vi "FPGA_Main.vi"() -> ()   [LabVIEW 2017]
doc: "Przekazywanie sygnału audio, o wybranej częstotliwości próbkowania, do FIFO. Vi ma za zadanie przeprowadzić pierwszą selekcję sygnałów, poprzez wprowadzenie odpowiedniego \"Thresholdu\", a następnie zebrania odpowiedniej ilości próbek, aby wysłać paczkę do RT."
uses:
  Custom Controls/#typedef_MicrophoneData.ctl
  <vilib>/LabVIEW Targets/FPGA/RIO/BlueMoonOnboardIO/nicrio_cRIO-BlueMoonOnboardAi_TerminalMod.ctl
  <vilib>/LabVIEW Targets/FPGA/RIO/BlueMoonOnboardIO/nicrio_cRIO-BlueMoonOnboardAi_VoltageRange.ctl
  <vilib>/rvi/Emulation/niFpgaGetClockAttributes.vi
  <vilib>/rvi/Emulation/niFpgaSctlEmulationGetInTimedLoop.vi
  <vilib>/rvi/Emulation/niFpgaEmulationReportErrorSimple.vi
  <vilib>/rvi/eio/common/nirviEmuTemplateMethod_errors.vi
  <vilib>/rvi/eio/common/nirviEmuTemplatePropertySet_noerrors.vi
  <vilib>/rvi/interface/RandomDataEmulation/niFpgaRandomDataHandleErrors.vi
  <vilib>/rvi/Emulation/niFpgaCriticalErrorInLSC.vi
  <vilib>/eio/EIONode/EIONode.xnode
  <vilib>/eio/EIOPropertyNode/EIOPropertyNode.xnode
  <vilib>/rvi/Analysis/measure/butterworth/XNode/niFpgaButterworthFilter.xnode
  <vilib>/rvi/DataTransferAndStorage/Container/XNode/niFpgaContainer.xnode
  <vilib>/rvi/interface/RandomDataEmulation/nirviRandomDataFpgaReadWriteTemplate.vi
  <vilib>/rvi/eio/common/nirviEmuTemplatePropertyGet_errors.vi
  <vilib>/rvi/eio/common/nirviEmuTemplatePropertyGet_noerrors.vi
  <vilib>/rvi/eio/common/nirviEmuTemplatePropertySet_errors.vi
panel:
  in  "SamplesToSend":u32
  in  "NoiseSamplesToReject":u32
  in  "Threshold":fxp<+/-,28,9>
  out "Mic_4_FIFO_Timed Out?":bool
  out "Mic_3_FIFO_Timed Out?":bool
  out "Mic_2_FIFO_Timed Out?":bool
  out "Mic_1_FIFO_Timed Out?":bool
  in  "AcqLoopDelay(uSec)":u32 caption="Count(uSec)"
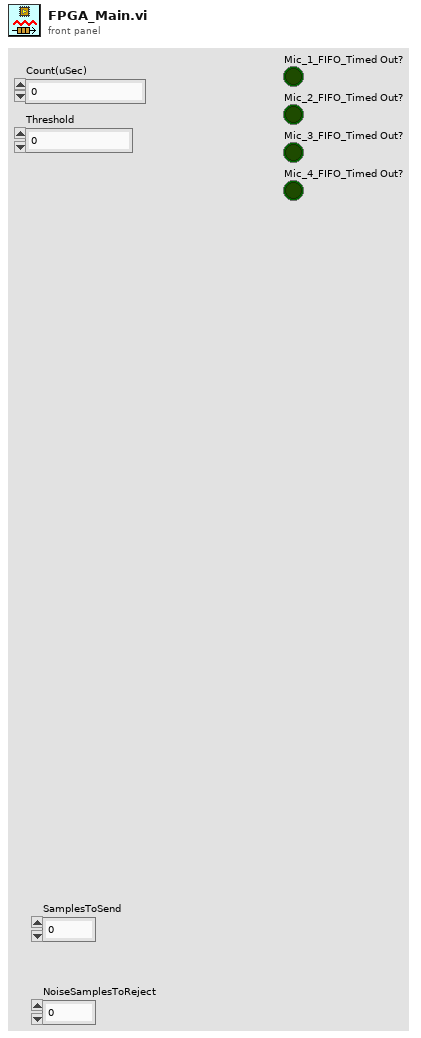
[diagram p1: front panel]
types:
  T1 = typedef "#typedef_MicrophoneData.ctl" = cluster{"output data":fxp<+/-,28,9>, "output data":fxp<+/-,28,9>, "output data":fxp<+/-,28,9>, "output data":fxp<+/-,28,9>}
  T2 = typedef "nicrio_cRIO-BlueMoonOnboardAi_VoltageRange.ctl" = u8
  T3 = typedef "nicrio_cRIO-BlueMoonOnboardAi_TerminalMod.ctl" = u8
  T4 = cluster{"output data":bool, "output data":bool, "output data":bool, "output data":bool}
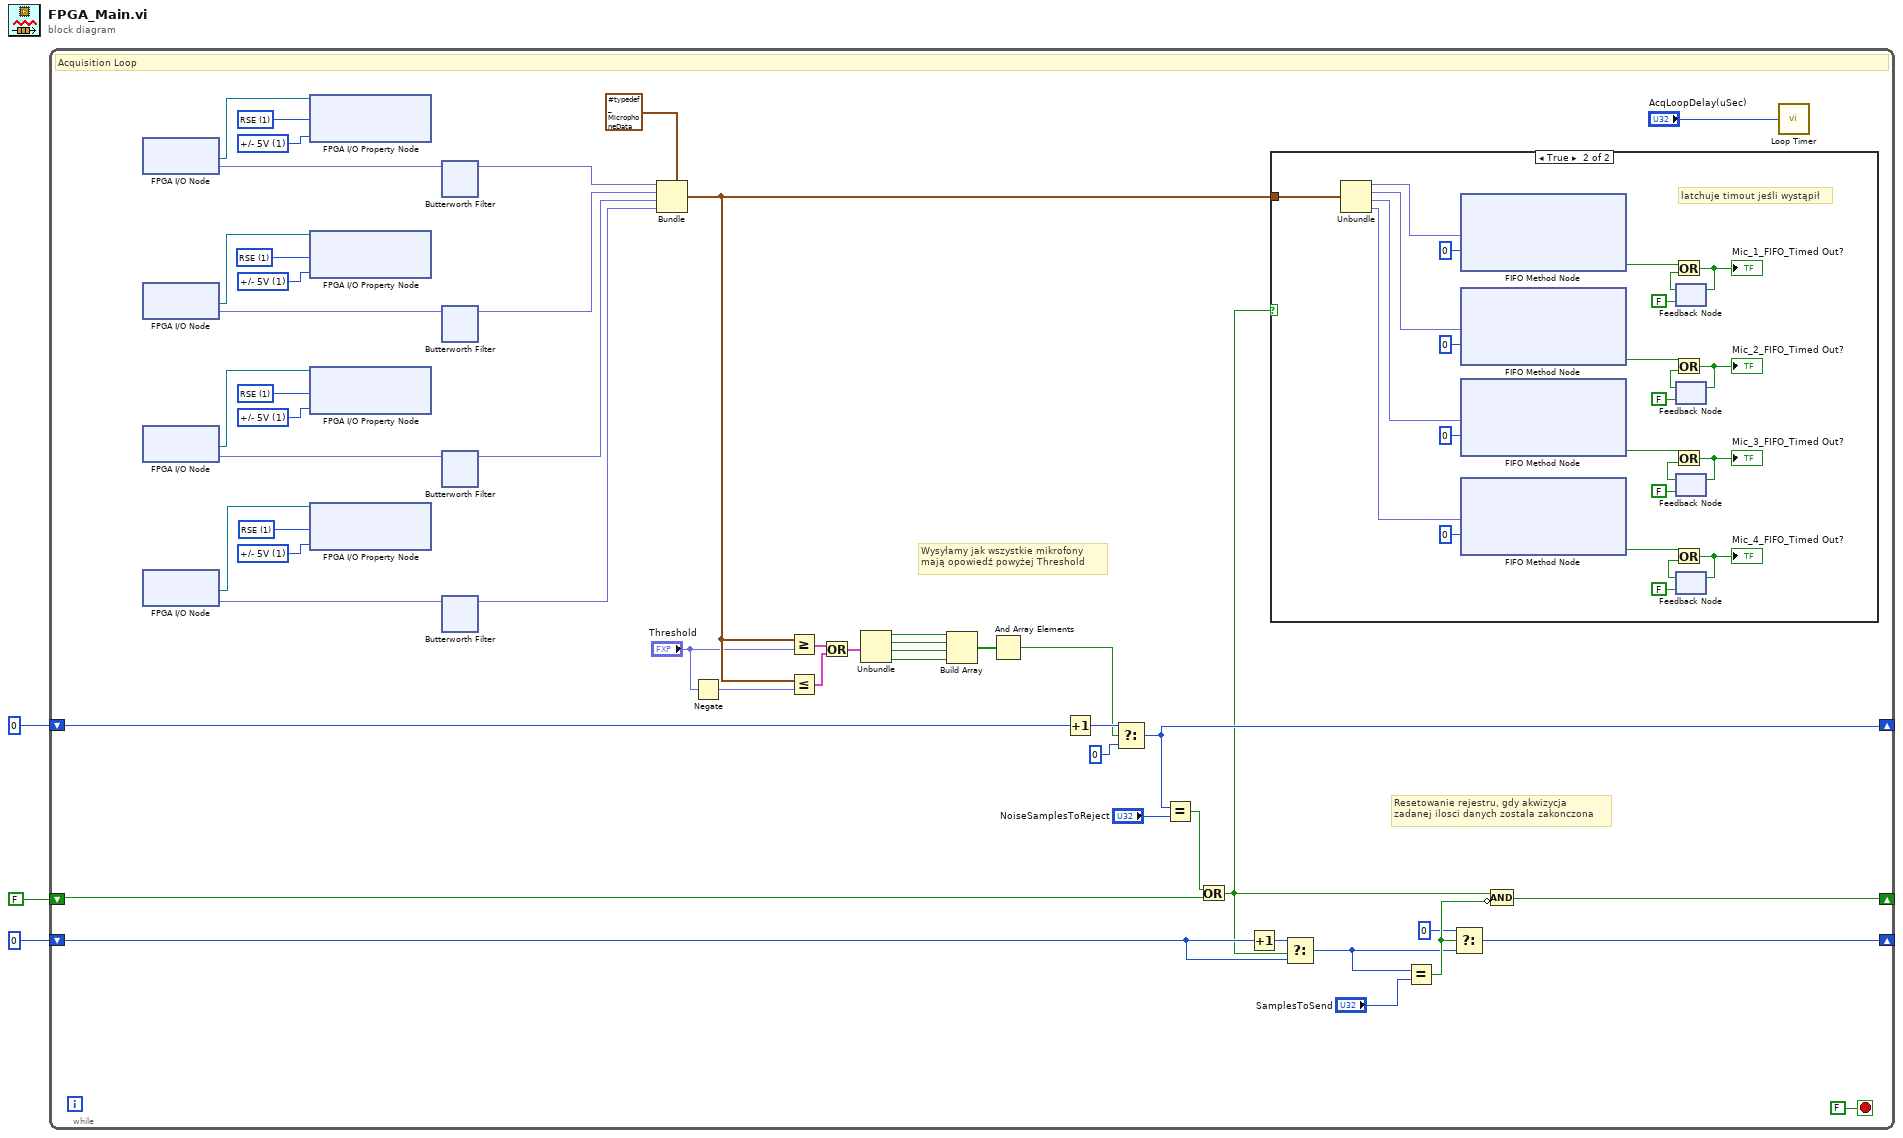
[diagram p0: block diagram]
diagram:
  n1 = while {
    shift-right: [w41] -> _
    shift-left: u32 0 -> [w44]
    shift-right: [w29] -> _
    shift-left: u32 0 -> [w28]
    shift-right: [w30] -> _
    shift-left: FALSE -> [w27]
    stop <- FALSE stop-if-true
    w7 = T2 1 items=["+/- 10V", "+/- 5V", "+/- 2V", "+/- 1V"] ("Voltage Range")
    w6 = T3 1 items=["DIFF", "RSE"] ("Terminal Mode")
    w9 = T2 1 items=["+/- 10V", "+/- 5V", "+/- 2V", "+/- 1V"] ("Voltage Range")
    w8 = T3 1 items=["DIFF", "RSE"] ("Terminal Mode")
    w11 = T2 1 items=["+/- 10V", "+/- 5V", "+/- 2V", "+/- 1V"] ("Voltage Range")
    w10 = T3 1 items=["DIFF", "RSE"] ("Terminal Mode")
    w12 = T2 1 items=["+/- 10V", "+/- 5V", "+/- 2V", "+/- 1V"] ("Voltage Range")
    w13 = T3 1 items=["DIFF", "RSE"] ("Terminal Mode")
    # "Wysyłamy jak wszystkie mikrofony \nmają opowiedź powyżej Threshold"
    # "Resetowanie rejestru, gdy akwizycja \nzadanej ilosci danych zostala zakonczona"
    # "Acquisition Loop"
    n2 = xnode "FPGA I/O Node"() -> ("Mic_1"=w51:fxp<+/-,24,5>, "FPGA I/O Out"=w14:refnum<k21>)  [unwired: 1 in]
    n3 = xnode "FPGA I/O Node"() -> ("Mic_2"=w52:fxp<+/-,24,5>, "FPGA I/O Out"=w15:refnum<k21>)  [unwired: 1 in]
    n4 = xnode "FPGA I/O Node"() -> ("Mic_3"=w53:fxp<+/-,24,5>, "FPGA I/O Out"=w16:refnum<k21>)  [unwired: 1 in]
    n5 = xnode "FPGA I/O Node"() -> ("Mic_4"=w50:fxp<+/-,24,5>, "FPGA I/O Out"=w17:refnum<k21>)  [unwired: 1 in]
    n6 = xnode "FPGA I/O Property Node"("FPGA I/O In"=w14, "Terminal Mode"=w6, "Voltage Range"=w7) -> ()  [unwired: 1 out]
    n7 = xnode "FPGA I/O Property Node"("FPGA I/O In"=w15, "Terminal Mode"=w8, "Voltage Range"=w9) -> ()  [unwired: 1 out]
    n8 = xnode "FPGA I/O Property Node"("FPGA I/O In"=w16, "Terminal Mode"=w10, "Voltage Range"=w11) -> ()  [unwired: 1 out]
    n9 = xnode "FPGA I/O Property Node"("FPGA I/O In"=w17, "Terminal Mode"=w13, "Voltage Range"=w12) -> ()  [unwired: 1 out]
    n10 = xnode "Butterworth Filter"("input data"=w51) -> ("output data"=w22:fxp<+/-,28,9>)  [unwired: 2 in]
    n11 = xnode "Butterworth Filter"("input data"=w52) -> ("output data"=w21:fxp<+/-,28,9>)  [unwired: 2 in]
    n12 = xnode "Butterworth Filter"("input data"=w53) -> ("output data"=w19:fxp<+/-,28,9>)  [unwired: 2 in]
    n13 = xnode "Butterworth Filter"("input data"=w50) -> ("output data"=w20:fxp<+/-,28,9>)  [unwired: 2 in]
    n14 = Bundle(cluster=T1 {"output data"=0.0, "output data"=0.0, "output data"=0.0, "output data"=0.0}, "output data"=w22, "output data"=w21, "output data"=w19, "output data"=w20) -> (w18:T1)
    n15 = Negate(x="Threshold") -> (-x=w4:fxp<+/-,28,9>)
    n16 = Greater Or Equal?(x=w18, y="Threshold") -> (x >= y?=w24:T4)
    n17 = Less Or Equal?(x=w18, y=w4) -> (x <= y?=w23:T4)
    n18 = Or(x=w24, y=w23) -> (x .or. y?=w25:T4)
    n19 = Unbundle(w25) -> ("output data"=w32:bool, "output data"=w33:bool, "output data"=w34:bool, "output data"=w31:bool)
    n20 = Build Array(w32, w33, w34, w31) -> (w47:bool[])
    n21 = And Array Elements(Boolean array=w47) -> (logical AND=w43:bool)
    n22 = Increment(x=w44) -> (x+1=w45:u32)
    n23 = Select(t=w45, s=w43, f=u32 0) -> (s? t:f=w41:u32)
    n24 = Equal?(x=w41, y="NoiseSamplesToReject") -> (x = y?=w35:bool)
    n25 = Or(x=w35, y=w27) -> (x .or. y?=w26:bool)
    n26 = Increment(x=w28) -> (x+1=w36:u32)
    n27 = case shown="True" w26 {
      tunnel: w18 -> [_ w111]
      frame False {
      }
      frame True {
        # "latchuje timout jeśli wystąpił"
        n28 = Unbundle(w111) -> ("output data"=w87:fxp<+/-,28,9>, "output data"=w108:fxp<+/-,28,9>, "output data"=w109:fxp<+/-,28,9>, "output data"=w110:fxp<+/-,28,9>)
        n29 = xnode ("FIFO Method Node")("Element"=w87, "Timeout"=0) -> ("Timed Out?"=w89:bool)  [unwired: 1 in, 1 out]
        n30 = xnode ("FIFO Method Node")("Element"=w108, "Timeout"=0) -> ("Timed Out?"=w93:bool)  [unwired: 1 in, 1 out]
        n31 = xnode ("FIFO Method Node")("Element"=w109, "Timeout"=0) -> ("Timed Out?"=w96:bool)  [unwired: 1 in, 1 out]
        n32 = xnode ("FIFO Method Node")("Element"=w110, "Timeout"=0) -> ("Timed Out?"=w100:bool)  [unwired: 1 in, 1 out]
        n33 = feedback #1(FALSE) -> (w91:bool)
        n34 = Or(x=w89, y=w91) -> (x .or. y?=w88:bool)
        "Mic_1_FIFO_Timed Out?" <- w88
        n35 = feedback-in #1(w88) -> ()
        n36 = feedback #2(FALSE) -> (w101:bool)
        n37 = Or(x=w93, y=w101) -> (x .or. y?=w92:bool)
        "Mic_2_FIFO_Timed Out?" <- w92
        n38 = feedback-in #2(w92) -> ()
        n39 = feedback #3(FALSE) -> (w103:bool)
        n40 = Or(x=w96, y=w103) -> (x .or. y?=w95:bool)
        "Mic_3_FIFO_Timed Out?" <- w95
        n41 = feedback-in #3(w95) -> ()
        n42 = feedback #4(FALSE) -> (w99:bool)
        n43 = Or(x=w100, y=w99) -> (x .or. y?=w98:bool)
        "Mic_4_FIFO_Timed Out?" <- w98
        n44 = feedback-in #4(w98) -> ()
      }
    }
    n45 = Select(t=w36, s=w26, f=w28) -> (s? t:f=w37:u32)
    n46 = Equal?(x=w37, y="SamplesToSend") -> (x = y?=w40:bool)
    n47 = Select(t=u32 0, s=w40, f=w37) -> (s? t:f=w29:u32)
    n48 = Compound Arithmetic op=AND(w26, invert w40) -> (w30:bool)
    n49 = call "Loop Timer"("Count(uSec)"="AcqLoopDelay(uSec)") -> ()  [unwired: 1 out]
  }
